vi "CIFreq.vi"(8 "error in (no error)":errorcluster, 11 "reference":refnum<k24>) -> (0 "error out":errorcluster, 1 "StartingEdge":i32(ring) items=["Rising", "Falling"], 2 "MeasurementTime":dbl, 3 "reference out":refnum<k24>, 4 "Units":i32(ring) items=["Hz", "Ticks"])   [LabVIEW 2009]
uses:
  C:/Program Files/National Instruments/LabVIEW 2009/vi.lib/ULx/ULx_LV.dll
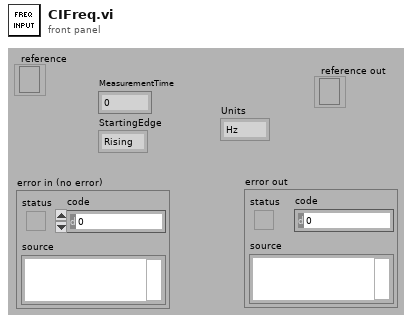
[diagram p1: front panel]
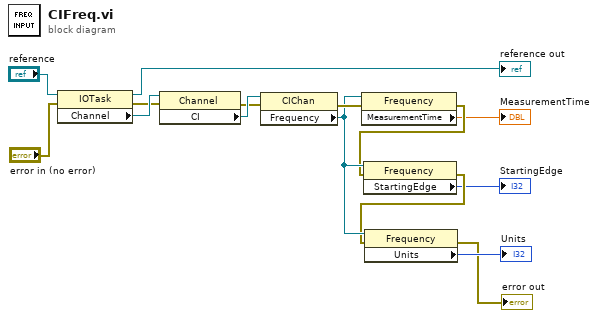
[diagram p0: block diagram]
diagram:
  n1 = property class="IOTask"(reference="reference", error in="error in (no error)") -> (reference out=→"reference out":refnum<k24>, error out=w12:errorcluster, "Channel"=w15:refnum<k24>)
  n2 = property class="Channel"(reference=w15, error in=w12) -> (error out=w11:errorcluster, "CI"=w14:refnum<k24>)  [unwired: 1 out]
  n3 = property class="CIChan"(reference=w14, error in=w11) -> (error out=w10:errorcluster, "Frequency"=w9:refnum<k24>)  [unwired: 1 out]
  n4 = property class="Frequency"(reference=w9, error in=w10) -> (error out=w8:errorcluster, "MeasurementTime"=→"MeasurementTime":dbl)  [unwired: 1 out]
  n5 = property class="Frequency"(reference=w9, error in=w8) -> (error out=w7:errorcluster, "StartingEdge"=→"StartingEdge":i32)  [unwired: 1 out]
  n6 = property class="Frequency"(reference=w9, error in=w7) -> (error out=→"error out":errorcluster, "Units"=→"Units":i32)  [unwired: 1 out]
